vi "To output format x410.vi"(8 "input valid":bool=TRUE, 10 "factor":u16, 11 "Data in":fxp<+/-,32,14>[](array[numeric])=[0.0, 0.0]) -> (0 "output valid":bool, 3 "Data out":T1)   [LabVIEW 2025]
uses:
  IQ-1element.ctl
  <instrlib>/_niInstr/DSP/v1/Shared/Public/IQ Data.ctl
  <vilib>/rvi/FXPMathLib/FxpConvert/subVIs/nifxpmath_Convert_SimConfig.ctl
  <vilib>/fxp/LVFixedPointQuantizationPolicyTypeDef.ctl
  <vilib>/fxp/LVFixedPointOverflowPolicyTypeDef.ctl
  <vilib>/rvi/FXPMathLib/FxpConvert/simVIs/DllFxpConvertTemp_sub.vi
  <vilib>/rvi/FXPMathLib/FxpInterpret/XNode/nifxpmath_Interpret.xnode
  <vilib>/rvi/FXPMathLib/FxpConvert/XNode/nifxpmath_Convert.xnode
  <instrlib>/_niInstr/DSP/v1/Shared/niInstr DSP v1 Shared.lvlib
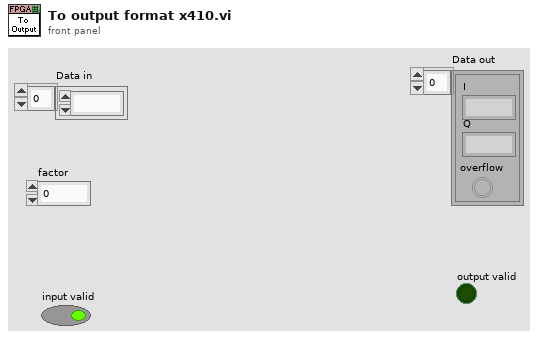
[diagram p1: front panel]
types:
  T1 = typedef "IQ-1element.ctl" = T2[]
  T2 = typedef "niInstr DSP v1 Shared.lvlib/IQ Data.ctl" = cluster{"I":fxp<+/-,18,1>, "Q":fxp<+/-,18,1>, "overflow":bool}
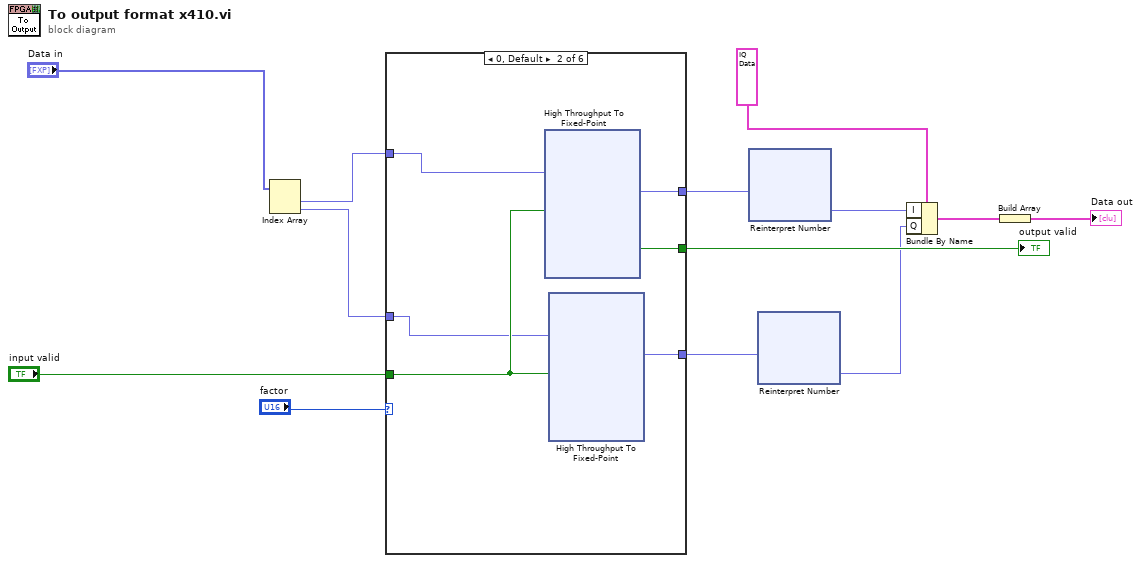
[diagram p0: block diagram]
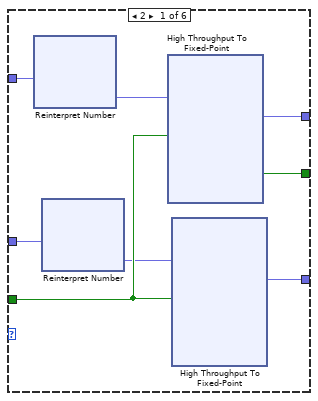
[diagram p2: hidden frame]
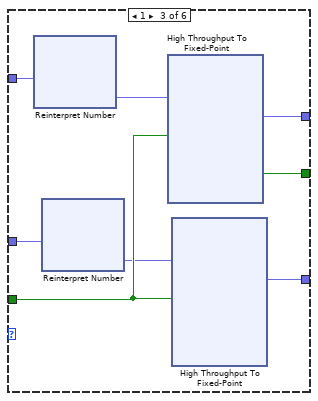
[diagram p3: hidden frame]
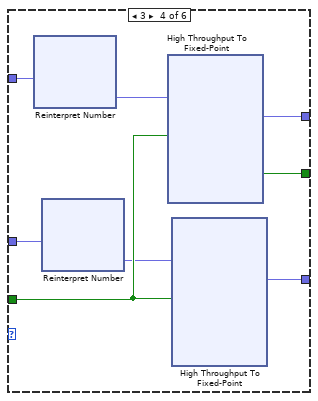
[diagram p4: hidden frame]
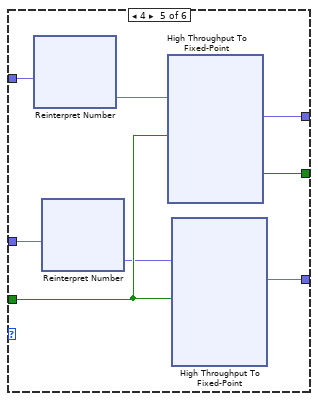
[diagram p5: hidden frame]
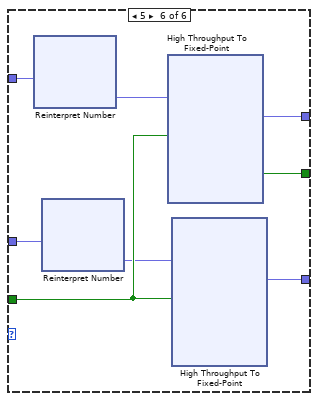
[diagram p6: hidden frame]
diagram:
  n1 = Index Array(array="Data in") -> (element #1=w10:fxp<+/-,32,14>, element #2=w9:fxp<+/-,32,14>)  [unwired: 2 in]
  n2 = case shown="0, Default" "factor" {
    tunnel: "input valid" -> [w21 w75 w131 w187 w243 w299]
    tunnel: [w20 w74 w130 w186 w242 w298] -> w12
    tunnel: [w19 w73 w129 w185 w241 w297] -> w4
    tunnel: [w18 w72 w128 w184 w240 w296] -> w2
    tunnel: w10 -> [w17 w71 w127 w183 w239 w295]
    tunnel: w9 -> [w15 w70 w125 w181 w237 w293]
    frame 2 {
      n3 = xnode "Reinterpret Number"("x"=w17) -> ("y"=w16:fxp<+/-,32,16>)
      n4 = xnode "Reinterpret Number"("x"=w15) -> ("y"=w14:fxp<+/-,32,16>)
      n5 = xnode "High Throughput To Fixed-Point"("x"=w16, "input valid"=w21) -> ("y"=w19:fxp<+/-,18,14>, "output valid"=w20:bool)  [unwired: 1 in, 1 out]
      n6 = xnode "High Throughput To Fixed-Point"("x"=w14, "input valid"=w21) -> ("y"=w18:fxp<+/-,18,14>)  [unwired: 1 in, 2 out]
    }
    frame 0, Default {
      n7 = xnode "High Throughput To Fixed-Point"("x"=w71, "input valid"=w75) -> ("y"=w73:fxp<+/-,18,14>, "output valid"=w74:bool)  [unwired: 1 in, 1 out]
      n8 = xnode "High Throughput To Fixed-Point"("x"=w70, "input valid"=w75) -> ("y"=w72:fxp<+/-,18,14>)  [unwired: 1 in, 2 out]
    }
    frame 1 {
      n9 = xnode "Reinterpret Number"("x"=w127) -> ("y"=w126:fxp<+/-,32,15>)
      n10 = xnode "Reinterpret Number"("x"=w125) -> ("y"=w124:fxp<+/-,32,15>)
      n11 = xnode "High Throughput To Fixed-Point"("x"=w126, "input valid"=w131) -> ("y"=w129:fxp<+/-,18,14>, "output valid"=w130:bool)  [unwired: 1 in, 1 out]
      n12 = xnode "High Throughput To Fixed-Point"("x"=w124, "input valid"=w131) -> ("y"=w128:fxp<+/-,18,14>)  [unwired: 1 in, 2 out]
    }
    frame 3 {
      n13 = xnode "Reinterpret Number"("x"=w183) -> ("y"=w182:fxp<+/-,32,17>)
      n14 = xnode "Reinterpret Number"("x"=w181) -> ("y"=w180:fxp<+/-,32,17>)
      n15 = xnode "High Throughput To Fixed-Point"("x"=w182, "input valid"=w187) -> ("y"=w185:fxp<+/-,18,14>, "output valid"=w186:bool)  [unwired: 1 in, 1 out]
      n16 = xnode "High Throughput To Fixed-Point"("x"=w180, "input valid"=w187) -> ("y"=w184:fxp<+/-,18,14>)  [unwired: 1 in, 2 out]
    }
    frame 4 {
      n17 = xnode "Reinterpret Number"("x"=w239) -> ("y"=w238:fxp<+/-,32,18>)
      n18 = xnode "Reinterpret Number"("x"=w237) -> ("y"=w236:fxp<+/-,32,18>)
      n19 = xnode "High Throughput To Fixed-Point"("x"=w238, "input valid"=w243) -> ("y"=w241:fxp<+/-,18,14>, "output valid"=w242:bool)  [unwired: 1 in, 1 out]
      n20 = xnode "High Throughput To Fixed-Point"("x"=w236, "input valid"=w243) -> ("y"=w240:fxp<+/-,18,14>)  [unwired: 1 in, 2 out]
    }
    frame 5 {
      n21 = xnode "Reinterpret Number"("x"=w295) -> ("y"=w294:fxp<+/-,32,19>)
      n22 = xnode "Reinterpret Number"("x"=w293) -> ("y"=w292:fxp<+/-,32,19>)
      n23 = xnode "High Throughput To Fixed-Point"("x"=w294, "input valid"=w299) -> ("y"=w297:fxp<+/-,18,14>, "output valid"=w298:bool)  [unwired: 1 in, 1 out]
      n24 = xnode "High Throughput To Fixed-Point"("x"=w292, "input valid"=w299) -> ("y"=w296:fxp<+/-,18,14>)  [unwired: 1 in, 2 out]
    }
  }
  "output valid" <- w12
  n25 = xnode "Reinterpret Number"("x"=w4) -> ("y"=w3:fxp<+/-,18,1>)
  n26 = xnode "Reinterpret Number"("x"=w2) -> ("y"=w1:fxp<+/-,18,1>)
  n27 = Bundle By Name(cluster=T2 {"I"=0.0, "Q"=0.0, "overflow"=FALSE} ("data"), "I"=w3, "Q"=w1) -> (w6:T2)
  n28 = Build Array(w6) -> (→"Data out":T2[])
